vi "2D sort.vi"(7 "Column Sort Order":i32[](array[numeric]), 11 "Array In":string[][](array[string])) -> (3 "Array Out":string[][](array[string]))   [LabVIEW 2014]
doc: "5/30/2001, Toby Stensland, toby@labjack.com, LabJack Corporation, www.labjack.com\n\nSorts a 2-dimensional array of strings. The number of columns in \"2D String Array In\" plus the number of elements in \"Column Sort Order\" must be less than or equal to 256.\n\n\"Ascending?\" -- Determines whether to sort data in ascending or descending order.\n\n\"Column Sort Order\" -- Number of elements of this array is between 0 and the number of columns of \"2D String Array In\". If this array is empty, the data is sorted by column 0, then 1, then 2, etc.\n\n\"2D String Array In\" -- 2-dimensional array of strings containing numbers, letters, and other."
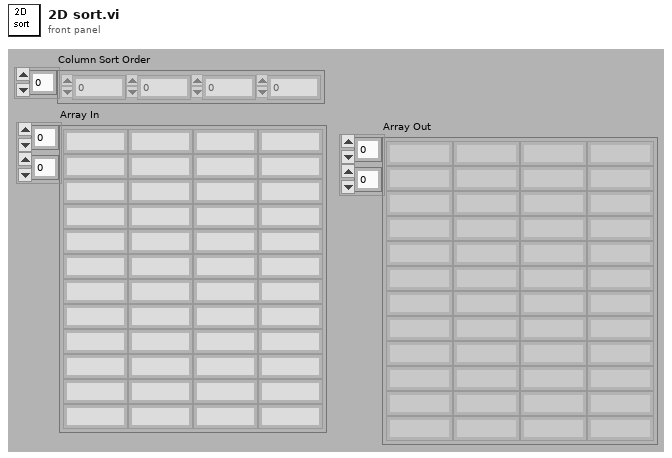
[diagram p1: front panel]
types:
  T1 = cluster{"Array In[0]":string, "Array In[1]":string, "Array In[2]":string, "Array In[3]":string, "Array In[4]":string, "Array In[5]":string, "Array In[6]":string, "Array In[7]":string, "Array In[8]":string, "Array In[9]":string, "Array In[10]":string, "Array In[11]":string, "Array In[12]":string, "Array In[13]":string, "Array In[14]":string, "Array In[15]":string, "Array In[16]":string, "Array In[17]":string, "Array In[18]":string, "Array In[19]":string, "Array In[20]":string, "Array In[21]":string, "Array In[22]":string, "Array In[23]":string, "Array In[24]":string, "Array In[25]":string, "Array In[26]":string, "Array In[27]":string, "Array In[28]":string, "Array In[29]":string, "Array In[30]":string, "Array In[31]":string, "Array In[32]":string, "Array In[33]":string, "Array In[34]":string, "Array In[35]":string, "Array In[36]":string, "Array In[37]":string, "Array In[38]":string, "Array In[39]":string, "Array In[40]":string, "Array In[41]":string, "Array In[42]":string, "Array In[43]":string, "Array In[44]":string, "Array In[45]":string, "Array In[46]":string, "Array In[47]":string, "Array In[48]":string, "Array In[49]":string, "Array In[50]":string, "Array In[51]":string, "Array In[52]":string, "Array In[53]":string, "Array In[54]":string, "Array In[55]":string, "Array In[56]":string, "Array In[57]":string, "Array In[58]":string, "Array In[59]":string, "Array In[60]":string, "Array In[61]":string, "Array In[62]":string, "Array In[63]":string, "Array In[64]":string, "Array In[65]":string, "Array In[66]":string, "Array In[67]":string, "Array In[68]":string, "Array In[69]":string, "Array In[70]":string, "Array In[71]":string, "Array In[72]":string, "Array In[73]":string, "Array In[74]":string, "Array In[75]":string, "Array In[76]":string, "Array In[77]":string, "Array In[78]":string, "Array In[79]":string, "Array In[80]":string, "Array In[81]":string, "Array In[82]":string, "Array In[83]":string, "Array In[84]":string, "Array In[85]":string, "Array In[86]":string, "Array In[87]":string, "Array In[88]":string, "Array In[89]":string, "Array In[90]":string, "Array In[91]":string, "Array In[92]":string, "Array In[93]":string, "Array In[94]":string, "Array In[95]":string, "Array In[96]":string, "Array In[97]":string, "Array In[98]":string, "Array In[99]":string, "Array In[100]":string, "Array In[101]":string, "Array In[102]":string, "Array In[103]":string, "Array In[104]":string, "Array In[105]":string, "Array In[106]":string, "Array In[107]":string, "Array In[108]":string, "Array In[109]":string, "Array In[110]":string, "Array In[111]":string, "Array In[112]":string, "Array In[113]":string, "Array In[114]":string, "Array In[115]":string, "Array In[116]":string, "Array In[117]":string, "Array In[118]":string, "Array In[119]":string, "Array In[120]":string, "Array In[121]":string, "Array In[122]":string, "Array In[123]":string, "Array In[124]":string, "Array In[125]":string, "Array In[126]":string, "Array In[127]":string, "Array In[128]":string, "Array In[129]":string, "Array In[130]":string, "Array In[131]":string, "Array In[132]":string, "Array In[133]":string, "Array In[134]":string, "Array In[135]":string, "Array In[136]":string, "Array In[137]":string, "Array In[138]":string, "Array In[139]":string, "Array In[140]":string, "Array In[141]":string, "Array In[142]":string, "Array In[143]":string, "Array In[144]":string, "Array In[145]":string, "Array In[146]":string, "Array In[147]":string, "Array In[148]":string, "Array In[149]":string, "Array In[150]":string, "Array In[151]":string, "Array In[152]":string, "Array In[153]":string, "Array In[154]":string, "Array In[155]":string, "Array In[156]":string, "Array In[157]":string, "Array In[158]":string, "Array In[159]":string, "Array In[160]":string, "Array In[161]":string, "Array In[162]":string, "Array In[163]":string, "Array In[164]":string, "Array In[165]":string, "Array In[166]":string, "Array In[167]":string, "Array In[168]":string, "Array In[169]":string, "Array In[170]":string, "Array In[171]":string, "Array In[172]":string, "Array In[173]":string, "Array In[174]":string, "Array In[175]":string, "Array In[176]":string, "Array In[177]":string, "Array In[178]":string, "Array In[179]":string, "Array In[180]":string, "Array In[181]":string, "Array In[182]":string, "Array In[183]":string, "Array In[184]":string, "Array In[185]":string, "Array In[186]":string, "Array In[187]":string, "Array In[188]":string, "Array In[189]":string, "Array In[190]":string, "Array In[191]":string, "Array In[192]":string, "Array In[193]":string, "Array In[194]":string, "Array In[195]":string, "Array In[196]":string, "Array In[197]":string, "Array In[198]":string, "Array In[199]":string, "Array In[200]":string, "Array In[201]":string, "Array In[202]":string, "Array In[203]":string, "Array In[204]":string, "Array In[205]":string, "Array In[206]":string, "Array In[207]":string, "Array In[208]":string, "Array In[209]":string, "Array In[210]":string, "Array In[211]":string, "Array In[212]":string, "Array In[213]":string, "Array In[214]":string, "Array In[215]":string, "Array In[216]":string, "Array In[217]":string, "Array In[218]":string, "Array In[219]":string, "Array In[220]":string, "Array In[221]":string, "Array In[222]":string, "Array In[223]":string, "Array In[224]":string, "Array In[225]":string, "Array In[226]":string, "Array In[227]":string, "Array In[228]":string, "Array In[229]":string, "Array In[230]":string, "Array In[231]":string, "Array In[232]":string, "Array In[233]":string, "Array In[234]":string, "Array In[235]":string, "Array In[236]":string, "Array In[237]":string, "Array In[238]":string, "Array In[239]":string, "Array In[240]":string, "Array In[241]":string, "Array In[242]":string, "Array In[243]":string, "Array In[244]":string, "Array In[245]":string, "Array In[246]":string, "Array In[247]":string, "Array In[248]":string, "Array In[249]":string, "Array In[250]":string, "Array In[251]":string, "Array In[252]":string, "Array In[253]":string, "Array In[254]":string, "Array In[255]":string}
  T2 = cluster{"Array In[0]":string, "Array In[1]":string, "Array In[2]":string, "Array In[3]":string, "Array In[4]":string, "Array In[5]":string, "Array In[6]":string, "Array In[7]":string, "Array In[8]":string, "Array In[9]":string, "Array In[10]":string, "Array In[11]":string, "Array In[12]":string, "Array In[13]":string, "Array In[14]":string, "Array In[15]":string, "Array In[16]":string, "Array In[17]":string, "Array In[18]":string, "Array In[19]":string, "Array In[20]":string, "Array In[21]":string, "Array In[22]":string, "Array In[23]":string, "Array In[24]":string, "Array In[25]":string, "Array In[26]":string, "Array In[27]":string, "Array In[28]":string, "Array In[29]":string, "Array In[30]":string, "Array In[31]":string, "Array In[32]":string, "Array In[33]":string, "Array In[34]":string, "Array In[35]":string, "Array In[36]":string, "Array In[37]":string, "Array In[38]":string, "Array In[39]":string, "Array In[40]":string, "Array In[41]":string, "Array In[42]":string, "Array In[43]":string, "Array In[44]":string, "Array In[45]":string, "Array In[46]":string, "Array In[47]":string, "Array In[48]":string, "Array In[49]":string, "Array In[50]":string, "Array In[51]":string, "Array In[52]":string, "Array In[53]":string, "Array In[54]":string, "Array In[55]":string, "Array In[56]":string, "Array In[57]":string, "Array In[58]":string, "Array In[59]":string, "Array In[60]":string, "Array In[61]":string, "Array In[62]":string, "Array In[63]":string, "Array In[64]":string, "Array In[65]":string, "Array In[66]":string, "Array In[67]":string, "Array In[68]":string, "Array In[69]":string, "Array In[70]":string, "Array In[71]":string, "Array In[72]":string, "Array In[73]":string, "Array In[74]":string, "Array In[75]":string, "Array In[76]":string, "Array In[77]":string, "Array In[78]":string, "Array In[79]":string, "Array In[80]":string, "Array In[81]":string, "Array In[82]":string, "Array In[83]":string, "Array In[84]":string, "Array In[85]":string, "Array In[86]":string, "Array In[87]":string, "Array In[88]":string, "Array In[89]":string, "Array In[90]":string, "Array In[91]":string, "Array In[92]":string, "Array In[93]":string, "Array In[94]":string, "Array In[95]":string, "Array In[96]":string, "Array In[97]":string, "Array In[98]":string, "Array In[99]":string, "Array In[100]":string, "Array In[101]":string, "Array In[102]":string, "Array In[103]":string, "Array In[104]":string, "Array In[105]":string, "Array In[106]":string, "Array In[107]":string, "Array In[108]":string, "Array In[109]":string, "Array In[110]":string, "Array In[111]":string, "Array In[112]":string, "Array In[113]":string, "Array In[114]":string, "Array In[115]":string, "Array In[116]":string, "Array In[117]":string, "Array In[118]":string, "Array In[119]":string, "Array In[120]":string, "Array In[121]":string, "Array In[122]":string, "Array In[123]":string, "Array In[124]":string, "Array In[125]":string, "Array In[126]":string, "Array In[127]":string, "Array In[128]":string, "Array In[129]":string, "Array In[130]":string, "Array In[131]":string, "Array In[132]":string, "Array In[133]":string, "Array In[134]":string, "Array In[135]":string, "Array In[136]":string, "Array In[137]":string, "Array In[138]":string, "Array In[139]":string, "Array In[140]":string, "Array In[141]":string, "Array In[142]":string, "Array In[143]":string, "Array In[144]":string, "Array In[145]":string, "Array In[146]":string, "Array In[147]":string, "Array In[148]":string, "Array In[149]":string, "Array In[150]":string, "Array In[151]":string, "Array In[152]":string, "Array In[153]":string, "Array In[154]":string, "Array In[155]":string, "Array In[156]":string, "Array In[157]":string, "Array In[158]":string, "Array In[159]":string, "Array In[160]":string, "Array In[161]":string, "Array In[162]":string, "Array In[163]":string, "Array In[164]":string, "Array In[165]":string, "Array In[166]":string, "Array In[167]":string, "Array In[168]":string, "Array In[169]":string, "Array In[170]":string, "Array In[171]":string, "Array In[172]":string, "Array In[173]":string, "Array In[174]":string, "Array In[175]":string, "Array In[176]":string, "Array In[177]":string, "Array In[178]":string, "Array In[179]":string, "Array In[180]":string, "Array In[181]":string, "Array In[182]":string, "Array In[183]":string, "Array In[184]":string, "Array In[185]":string, "Array In[186]":string, "Array In[187]":string, "Array In[188]":string, "Array In[189]":string, "Array In[190]":string, "Array In[191]":string, "Array In[192]":string, "Array In[193]":string, "Array In[194]":string, "Array In[195]":string, "Array In[196]":string, "Array In[197]":string, "Array In[198]":string, "Array In[199]":string, "Array In[200]":string, "Array In[201]":string, "Array In[202]":string, "Array In[203]":string, "Array In[204]":string, "Array In[205]":string, "Array In[206]":string, "Array In[207]":string, "Array In[208]":string, "Array In[209]":string, "Array In[210]":string, "Array In[211]":string, "Array In[212]":string, "Array In[213]":string, "Array In[214]":string, "Array In[215]":string, "Array In[216]":string, "Array In[217]":string, "Array In[218]":string, "Array In[219]":string, "Array In[220]":string, "Array In[221]":string, "Array In[222]":string, "Array In[223]":string, "Array In[224]":string, "Array In[225]":string, "Array In[226]":string, "Array In[227]":string, "Array In[228]":string, "Array In[229]":string, "Array In[230]":string, "Array In[231]":string, "Array In[232]":string, "Array In[233]":string, "Array In[234]":string, "Array In[235]":string, "Array In[236]":string, "Array In[237]":string, "Array In[238]":string, "Array In[239]":string, "Array In[240]":string, "Array In[241]":string, "Array In[242]":string, "Array In[243]":string, "Array In[244]":string, "Array In[245]":string, "Array In[246]":string, "Array In[247]":string, "Array In[248]":string, "Array In[249]":string, "Array In[250]":string, "Array In[251]":string, "Array In[252]":string, "Array In[253]":string, "Array In[254]":string, "Array In[255]":string}[]
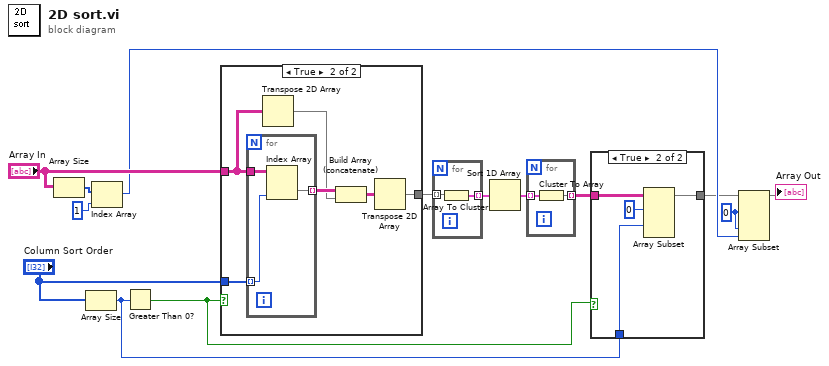
[diagram p0: block diagram]
diagram:
  w3 = 0 ("Array Index")
  n1 = Array Size(array="Array In") -> (size(s)=w11:i32[])
  n2 = Array Size(array="Column Sort Order") -> (size(s)=w9:i32)
  n3 = Index Array(array=w11, index=1 ("Index")) -> (element=w8:i32)
  n4 = Greater Than 0?(x=w9) -> (x > 0?=w13:bool)
  n5 = case shown="True" w13 {
    tunnel: "Column Sort Order" -> [_ w21]
    tunnel: "Array In" -> [w15 w20]
    tunnel: [w15 w16] -> w4
    frame False {
    }
    frame True {
      n6 = for {
        tunnel: w21 -> [w23] mode=indexing
        tunnel: w20 -> [w24]
        tunnel: [w22] -> w19 mode=indexing
        n7 = Index Array(array=w24, index (col)=w23) -> (element=w22:string[])  [unwired: 1 in]
      }
      n8 = Transpose 2D Array(2D array=w20) -> (transposed array=w18:string[][])
      n9 = Build Array (concatenate)(w19, w18) -> (w17:string[][])
      n10 = Transpose 2D Array(2D array=w17) -> (transposed array=w16:string[][])
    }
  }
  n11 = for {
    tunnel: w4 -> [w26] mode=indexing
    tunnel: [w25] -> w6 mode=indexing
    n12 = Array To Cluster(array=w26) -> (cluster=w25:T1)
  }
  n13 = Sort 1D Array(array=w6) -> (sorted array=w5:T2)
  n14 = for {
    tunnel: w5 -> [w28] mode=indexing
    tunnel: [w27] -> w2 mode=indexing
    n15 = Cluster To Array(cluster=w28) -> (array=w27:string[])
  }
  n16 = case shown="True" w13 {
    tunnel: [w29 w30] -> w1
    tunnel: w2 -> [w29 w33]
    tunnel: w9 -> [_ w32]
    frame False {
    }
    frame True {
      n17 = Array Subset(array=w33, index (row)=0 ("Array Index"), index (col)=w32) -> (w30:string[][])  [unwired: 2 in]
    }
  }
  n18 = Array Subset(array=w1, index (row)=w3, index (col)=w3, length (col)=w8) -> (→"Array Out":string[][])  [unwired: 1 in]
